vi "ReadFromArduino.vi"() -> ()   [LabVIEW 2018]
uses:
  <vilib>/Instr/_visa.llb/VISA Configure Serial Port (Instr).vi
panel:
  out "Cap_4":dbl(graph)
  out "Cap_3":dbl(graph)
  out "Cap_2":dbl(graph)
  out "Cap_1":dbl(graph)
  out "Read":i32(graph)
  in  "VISA resource name":refnum<visa-resource-name>
  in  "file (use dialog)":path=path "C:/Users/labadmin/Downloads/Testing.txt"
  in  "Save TEXT?":bool
  out "read":string
  in  "stop":bool
  out "Signal":dbl(graph)
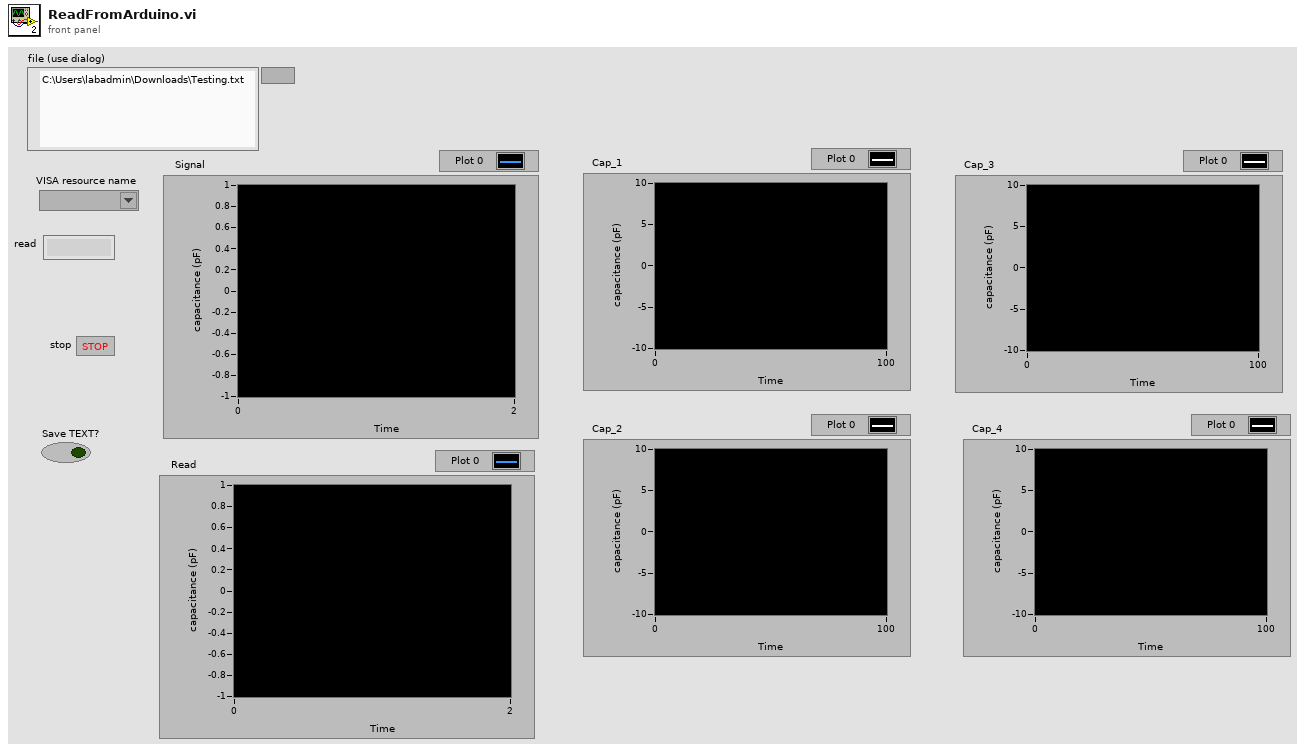
[diagram p1: front panel]
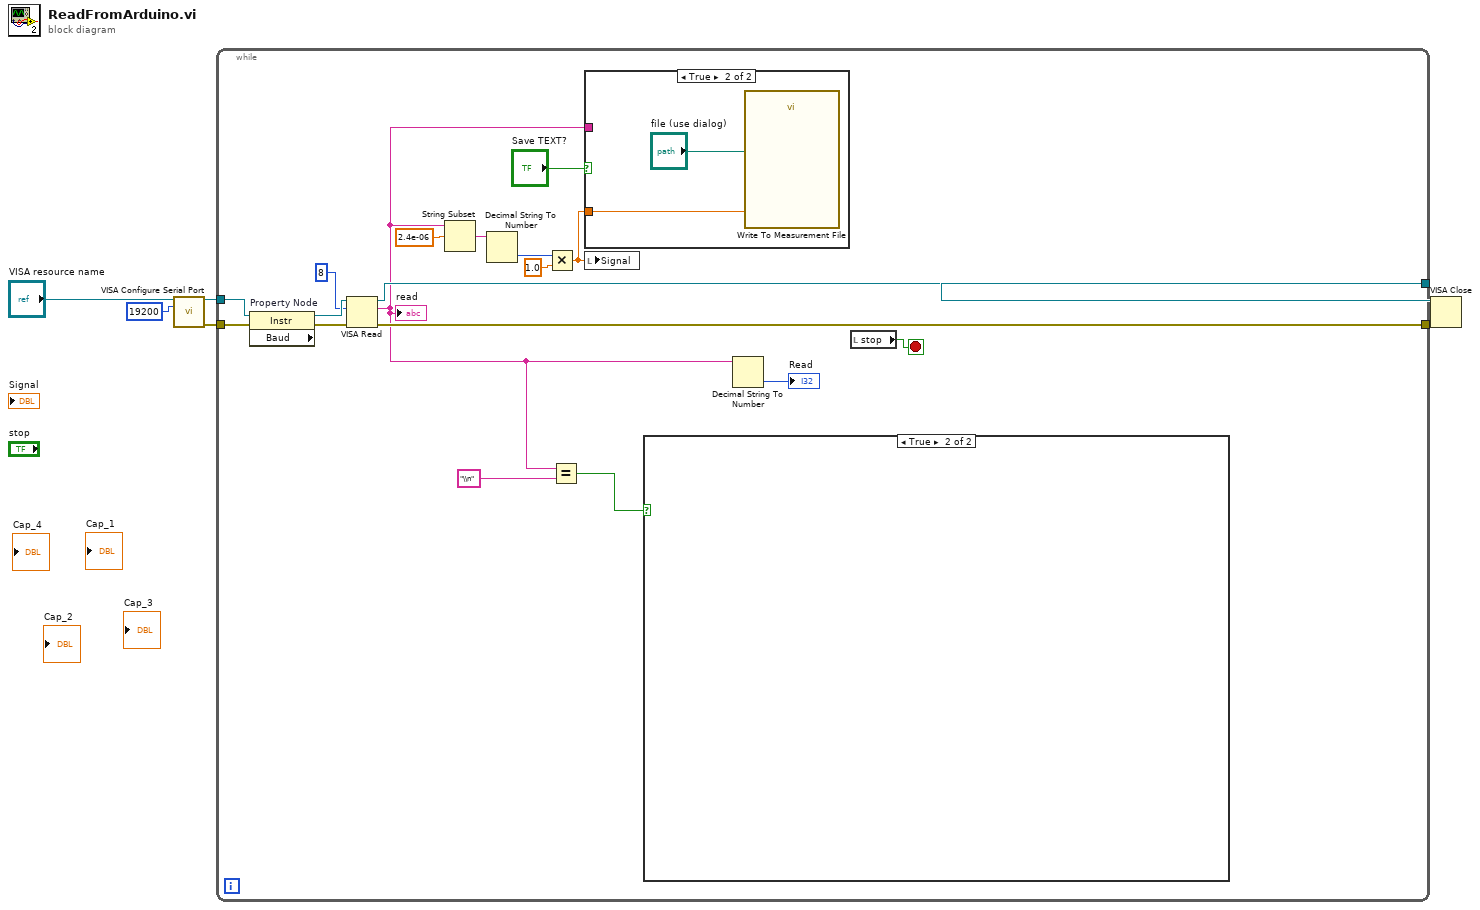
[diagram p0: block diagram]
diagram:
  n1 = call-poly "VISA Configure Serial Port"("VISA resource name"="VISA resource name", "baud rate (9600)"=u32 19200) -> ("VISA resource name out"=w4:refnum<visa-resource-name>, "error out"=w3:errorcluster)  [unwired: 12 in]
  n2 = while {
    tunnel: [w24] -> w6
    tunnel: [w23] -> w5
    tunnel: w4 -> [w22]
    tunnel: w3 -> [w21]
    stop <- w20 stop-if-true
    n3 = property on="Property Node" class="Instr" props=["Baud"](reference=w22, error in=w21) -> (reference out=w18:refnum<visa-resource-name>, error out=w19:errorcluster)  [unwired: 1 out]
    n4 = VISA Read(VISA resource name=w18, byte count=u32 8, error in (no error)=w19) -> (VISA resource name out=w24:refnum<visa-resource-name>, read buffer=w7:string, error out=w23:errorcluster)  [unwired: 1 out]
    "read" <- w7
    n5 = String Subset(string=w7, offset (0)=2.4e-06) -> (substring=w17:string)  [unwired: 1 in]
    n6 = Decimal String To Number(string=w17) -> (number=w15:i32)  [unwired: 2 in, 1 out]
    n7 = Multiply(x=w15, y=1.0 ("x")) -> (x*y=w11:dbl)
    n8 = Equal?(x=w7, y="\\n") -> (x = y?=w8:bool)
    n9 = case shown="True" "Save TEXT?" {
      tunnel: w7 -> [_ _]
      tunnel: w11 -> [_ w26]
      frame False {
      }
      frame True {
        n10 = call "Write To Measurement File"("Signals"=w26, "Filename"="file (use dialog)") -> ()  [unwired: 15 in, 3 out]
      }
    }
    n11 = local write "Signal"(w11) -> ()
    n12 = case shown="True" w8 {
      frame False {
      }
      frame True {
      }
    }
    n13 = Decimal String To Number(string=w7) -> (number=→"Read":i32)  [unwired: 2 in, 1 out]
    n14 = local read "stop"() -> (w20:bool)
  }
  n15 = VISA Close(VISA resource name=w6, error in (no error)=w5) -> ()  [unwired: 1 out]
